vi "F020_config_visa.vi"(8 "error in (no error)":errorcluster, 11 "VISA Refnum in":refnum<visa-resource-name>) -> (0 "error out":errorcluster, 3 "VISA Refnum out":refnum<visa-resource-name>)   [LabVIEW 2016]
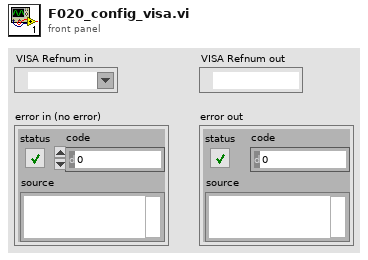
[diagram p1: front panel]
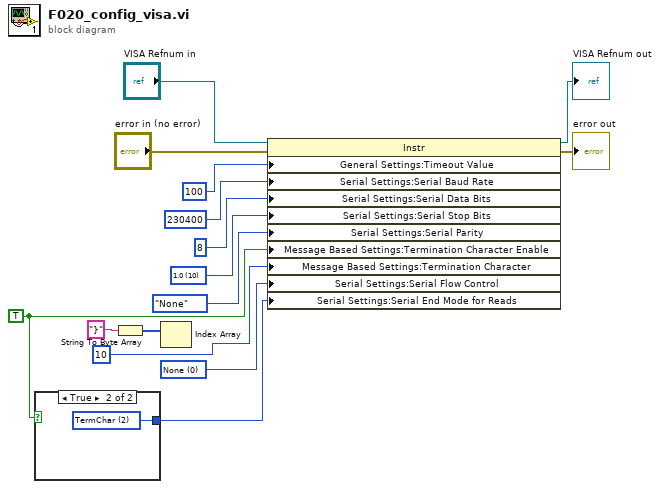
[diagram p0: block diagram]
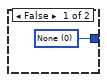
[diagram p2: hidden frame]
diagram:
  w12 = TRUE ("Enable Termination\nChar (T)")
  w13 = u16 0 items=["None", "XON/XOFF", "RTS/CTS", "XON/XOFF & RTS/CTS", "DTR/DSR", "XON/XOFF & DTR/DSR"] ("flow control (0:none)")
  w10 = u16 10 items=["1.0"=10, "1.5"=15, "2.0"=20] ("stop bits (10: 1 bit)")
  n1 = case shown="True" w12 {
    tunnel: [w16 w17] -> w11
    frame False {
      w16 = u16 0 items=["None", "LastBit", "TermChar"] ("Serial Settings:Serial End Mode for Reads")
    }
    frame True {
      w17 = u16 2 items=["None", "LastBit", "TermChar"] ("Serial Settings:Serial End Mode for Reads")
    }
  }
  n2 = String To Byte Array(string="}") -> (unsigned byte array=w15:u8[])
  n3 = Index Array(array=w15) -> ()  [unwired: 1 in, 1 out]
  n4 = property class="Instr"(reference="VISA Refnum in", error in="error in (no error)", "General Settings:Timeout Value"=u32 100 ("timeout (10sec)"), "Serial Settings:Serial Baud Rate"=u32 230400 ("baud rate (9600)"), "Serial Settings:Serial Data Bits"=u16 8 ("data bits (8)"), "Serial Settings:Serial Stop Bits"=w10, "Serial Settings:Serial Parity"=enum16{"None", "Odd", "Even", "Mark", "Space"}."None" ("parity (0:none)"), "Message Based Settings:Termination Character Enable"=w12, "Message Based Settings:Termination Character"=u8 10 ("element"), "Serial Settings:Serial Flow Control"=w13, "Serial Settings:Serial End Mode for Reads"=w11) -> (reference out=→"VISA Refnum out":refnum<visa-resource-name>, error out=→"error out":errorcluster)
